vi "RT.vi"() -> ()   [LabVIEW 2015]
uses:
  Types/RT Loop Events.ctl
panel:
  out "Connected":bool
  out "Error Out":errorcluster
  in  "Error In":errorcluster
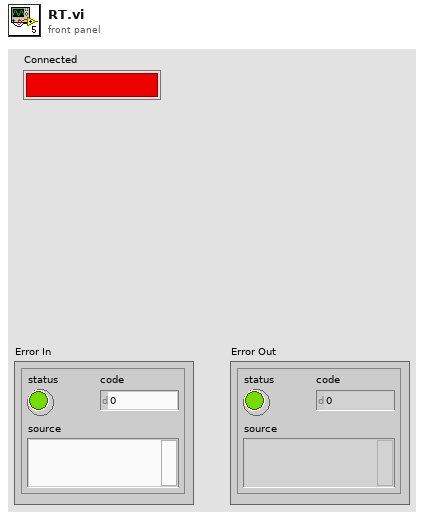
[diagram p1: front panel]
types:
  T1 = typedef "RT Loop Events.ctl" = enum16{"Initialize", "Wait for Connection", "Wait for Command", "Send Reply"}
  T2 = cluster{"RT Loop Events":T1, "Connection ID":refnum<k5>, "Message Data":string, "error constant":errorcluster}
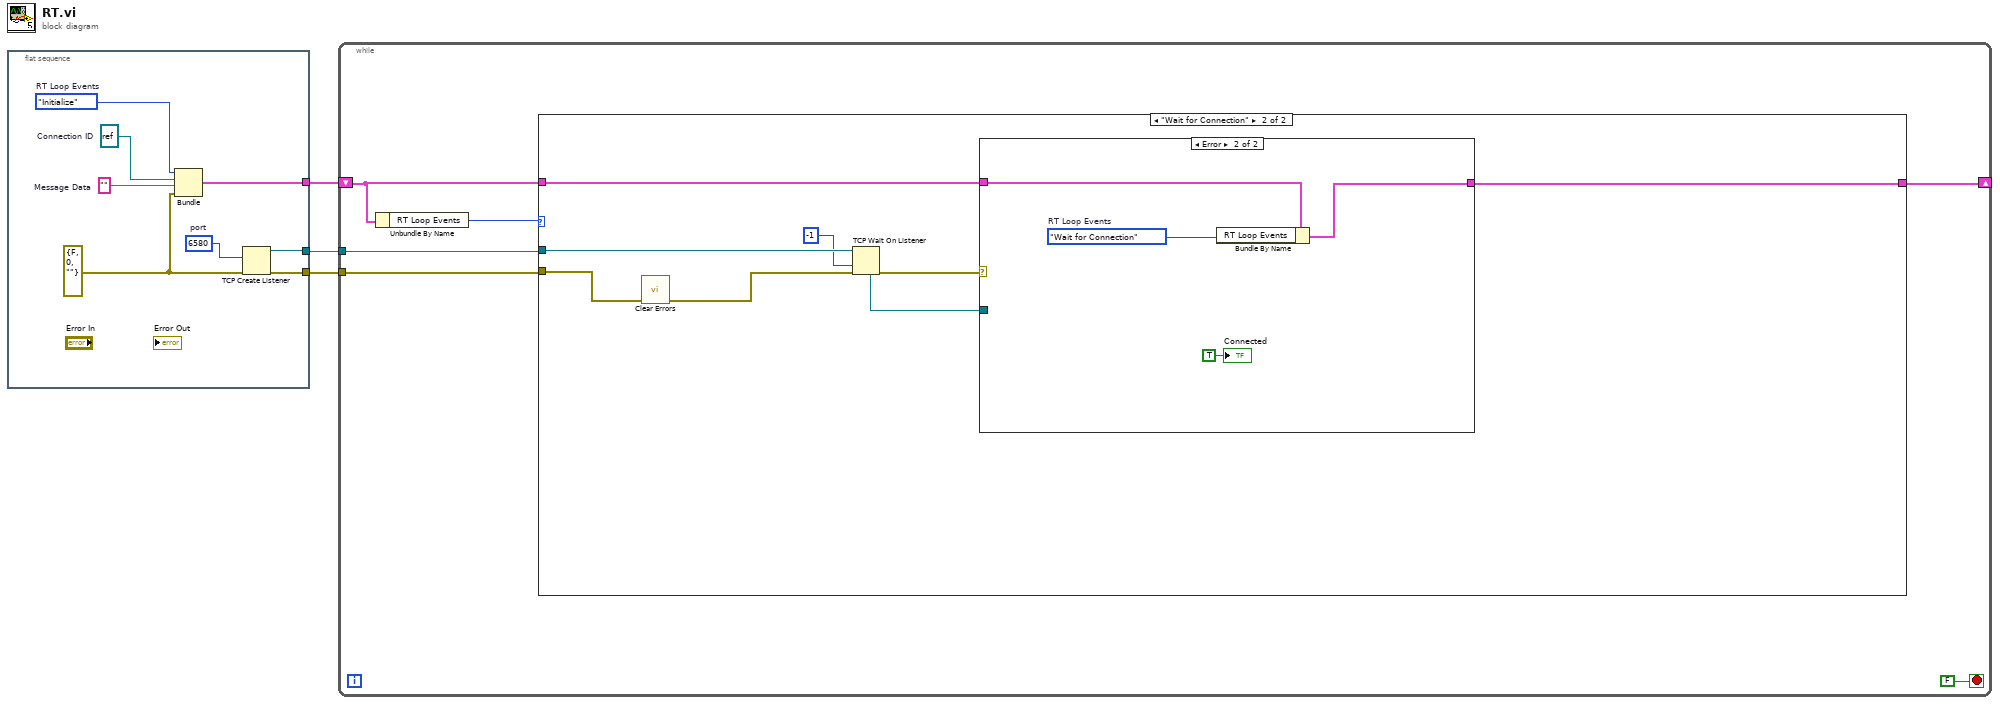
[diagram p0: block diagram]
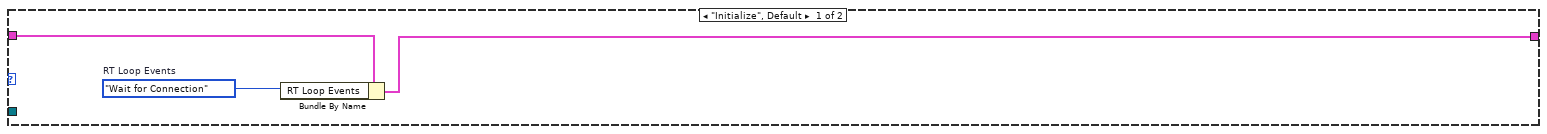
[diagram p2: hidden frame]
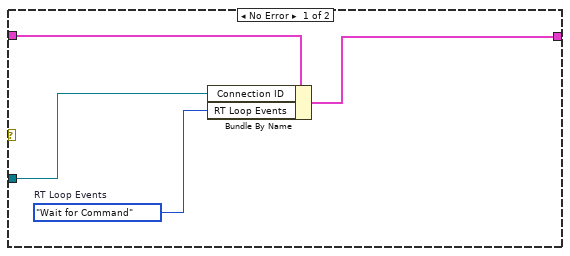
[diagram p3: hidden frame]
diagram:
  n1 = flat-sequence {
    tunnel: [w9] -> w3
    tunnel: [w6] -> w2
    tunnel: [w5] -> w1
    frame #0 {
      w4 = RT_Loop_Events."Initialize"  # RT Loop Events
      w8 = u16 6580  # port
      w11 = refnum<k5> refnum  # Connection ID
      w10 = ""  # Message Data
      w7 = errorcluster {"status"=FALSE, "code"=0, "source"=""} ("error constant")
      n2 = Bundle("RT Loop Events"=w4, "Connection ID"=w11, "Message Data"=w10, "error constant"=w7) -> (w9:T2)  [unwired: 1 in]
      n3 = TCP Create Listener(8:w7, 10:w8) -> (0:w5:errorcluster, 3:w6:refnum<k5>)  [unwired: 4 out]
    }
  }
  n4 = while {
    shift-right: [w12] -> _
    shift-left: w3 -> [w14]
    tunnel: w2 -> [w16]
    tunnel: w1 -> [w15]
    stop <- FALSE stop-if-true
    n5 = Unbundle By Name(w14) -> ("RT Loop Events"=w13:T1)
    n6 = case shown="\"Wait for Connection\"" w13 {
      tunnel: w16 -> [_ w27]
      tunnel: w15 -> [_ w28]
      tunnel: w14 -> [w20 w22]
      tunnel: [w19 w21] -> w12
      frame "Initialize", Default {
        w18 = RT_Loop_Events."Wait for Connection"  # RT Loop Events
        n7 = Bundle By Name(cluster=w20, "RT Loop Events"=w18) -> (w19:T2)
      }
      frame "Wait for Connection" {
        n8 = call <vilib>:"Clear Errors.vi"("error in (no error)"=w28) -> ("error out"=w25:errorcluster)  [unwired: 5 in, 1 out]
        n9 = TCP Wait On Listener(8:w25, 9:-1 ("timeout ms (wait forever: -1)"), 11:w27) -> (0:w24:errorcluster, 4:w23:refnum<k5>)  [unwired: 4 out]
        n10 = case shown="Error" w24 {
          tunnel: w23 -> [w30 _]
          tunnel: w22 -> [w32 w36]
          tunnel: [w31 w35] -> w21
          frame No Error {
            w29 = RT_Loop_Events."Wait for Command"  # RT Loop Events
            n11 = Bundle By Name(cluster=w32, "Connection ID"=w30, "RT Loop Events"=w29) -> (w31:T2)
          }
          frame Error {
            w34 = RT_Loop_Events."Wait for Connection"  # RT Loop Events
            n12 = Bundle By Name(cluster=w36, "RT Loop Events"=w34) -> (w35:T2)
            "Connected" <- TRUE ("Connected")
          }
        }
      }
    }
  }
